vi "ConcatenateWithReturn.vi"(5 "baseString":string, 9 "additionalString":string) -> (8 "outputString":string)   [LabVIEW 2016]
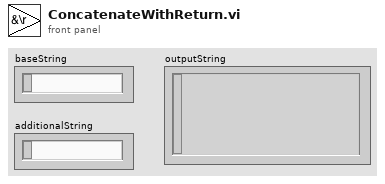
[diagram p1: front panel]
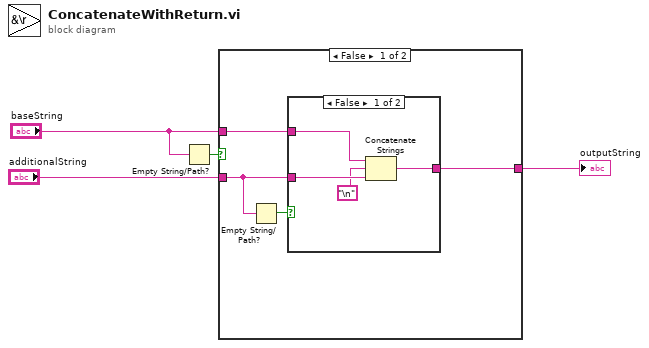
[diagram p0: block diagram]
diagram:
  n1 = Empty String/Path?(string/path="baseString") -> (empty?=w4:bool)
  n2 = case shown="False" w4 {
    tunnel: "additionalString" -> [w5 w14]
    tunnel: [w8 w14] -> w2
    tunnel: "baseString" -> [w7 _]
    frame False {
      n3 = Empty String/Path?(string/path=w5) -> (empty?=w6:bool)
      n4 = case shown="False" w6 {
        tunnel: w5 -> [w12 _]
        tunnel: [w11 w13] -> w8
        tunnel: w7 -> [w9 w13]
        frame False {
          n5 = Concatenate Strings(w9, "\n", w12) -> (w11:string)
        }
        frame True {
        }
      }
    }
    frame True {
    }
  }
  "outputString" <- w2
